vi "Reduce Fs.vi"(8 "error in (no error)":errorcluster, 11 "Instrument.DAQ in":refnum<class "Instrument.DAQ.lvclass">) -> (0 "error out":errorcluster, 3 "Instrument.DAQ out":refnum<class "Instrument.DAQ.lvclass">)   [LabVIEW 2019, in "Instrument.Lockin.lvlib" / "Instrument.DAQ.lvclass"]
uses:
  Instrument.DAQ.lvclass
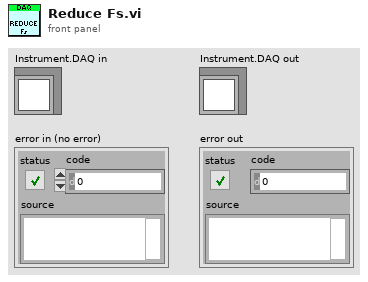
[diagram p1: front panel]
types:
  T1 = typedef "Instrument.Lockin.lvlib/Instrument.DAQ.lvclass/DAQ.Sampling--Cluster.ctl" = cluster{"Sampling":T2, "sample mode":i32, "Fs Mode":T3, "Fs Multiplier":dbl, "Refresh Rate (Hz)":dbl, "Decimation.PreDSP":i32, "Decimation.PostDSP":i32, "Fs.Output":dbl}
  T2 = typedef "Instrument.Lockin.lvlib/Instrument.DAQ.lvclass/DAQ.Sampling.Sampling--Cluster.ctl" = cluster{"Fs":dbl, "#s":i32}
  T3 = typedef "Instrument.Lockin.lvlib/Instrument.DAQ.lvclass/DAQ.Sampling.Fs Mode--enum.ctl" = enum16{"Manual", "Auto Fs", "Max Fs"}
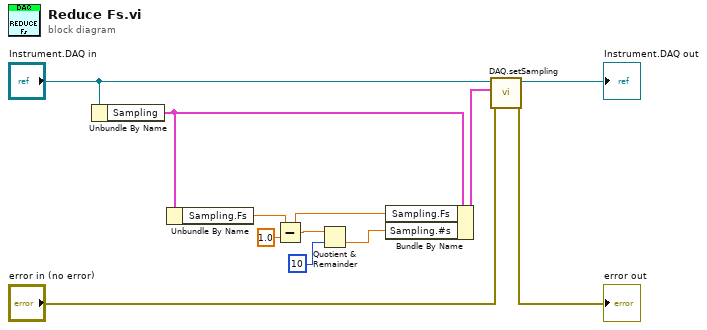
[diagram p0: block diagram]
diagram:
  n1 = Unbundle By Name("Instrument.DAQ in") -> ("Sampling"=w2:T1)
  n2 = Unbundle By Name(w2) -> ("Sampling.Fs"=w4:dbl)
  n3 = Subtract(x=w4, y=1.0) -> (x-y=w5:dbl)
  n4 = Quotient & Remainder(x=w5, y=10) -> (floor(x/y)=w6:dbl)  [unwired: 1 out]
  n5 = Bundle By Name(cluster=w2, "Sampling.Fs"=w5, "Sampling.#s"=w6) -> (w7:T1)
  n6 = call "DAQ.setSampling.vi"("error in (no error)"="error in (no error)", "Sampling"=w7, "Instrument.DAQ"="Instrument.DAQ in") -> ("error out"=→"error out":errorcluster, "Instrument.DAQ out"=→"Instrument.DAQ out":refnum<class "Instrument.DAQ.lvclass">)  [unwired: 7 in]
